vi "test-linear-filter-assert-results.vi"(5 "derivative":i32, 6 "Max":dbl, 7 "Samples":i32, 8 "Min":dbl, 9 "H":dbl, 10 "DerivFunc":refnum<vi>, 11 "F":refnum<vi>) -> (0 "Filt":dbl[](array[numeric]), 1 "Deriv":dbl[](array[numeric]), 2 "Raw":dbl[](array[numeric]), 3 "Passed":bool, 4 "Tolerance":dbl)   [LabVIEW 2019]
uses:
  <vilib>/Rock Robotics/WPI/ThirdParty/JAS_Junk/TrajLib/Matrix_Create.vi
  <vilib>/Rock Robotics/WPI/ThirdParty/JAS_Junk/TrajLib/LinearFilter_Factorial.vi
  <vilib>/Rock Robotics/WPI/ThirdParty/JAS_Junk/TrajLib/LinearFilter_New.vi
  <vilib>/Rock Robotics/WPI/ThirdParty/JAS_Junk/TrajLib/MatBuilder_Create.vi
  <vilib>/gmath/SpecialFunctions.llb/Factorial.vi
  <vilib>/Rock Robotics/SystemInterfaces/NetworkCommunication/NetComm_UsageReport_report.vi
  <vilib>/Analysis/7linalg.llb/Solve Linear Equations.vi
  <vilib>/Analysis/7linalg.llb/Solve Linear Equations (multiple right hand).vi
  <vilib>/Rock Robotics/WPI/ThirdParty/JAS_Junk/TrajLib/Util_LibraryGlobals.vi
  <vilib>/Rock Robotics/WPI/ThirdParty/JAS_Junk/TrajLib/Trajectory_Library.lvlib
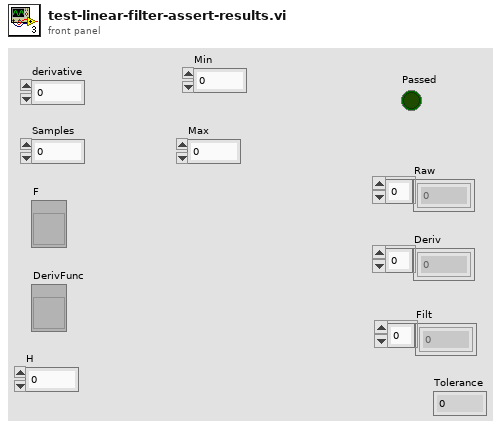
[diagram p1: front panel]
types:
  T1 = typedef "Trajectory_Library.lvlib/LINEAR_FILTER.ctl" = cluster{"InputGains":dbl[], "OutputGains":dbl[], "Inputs":dbl[], "Outputs":dbl[], "InGainCount":i32, "OutGainCount":i32}
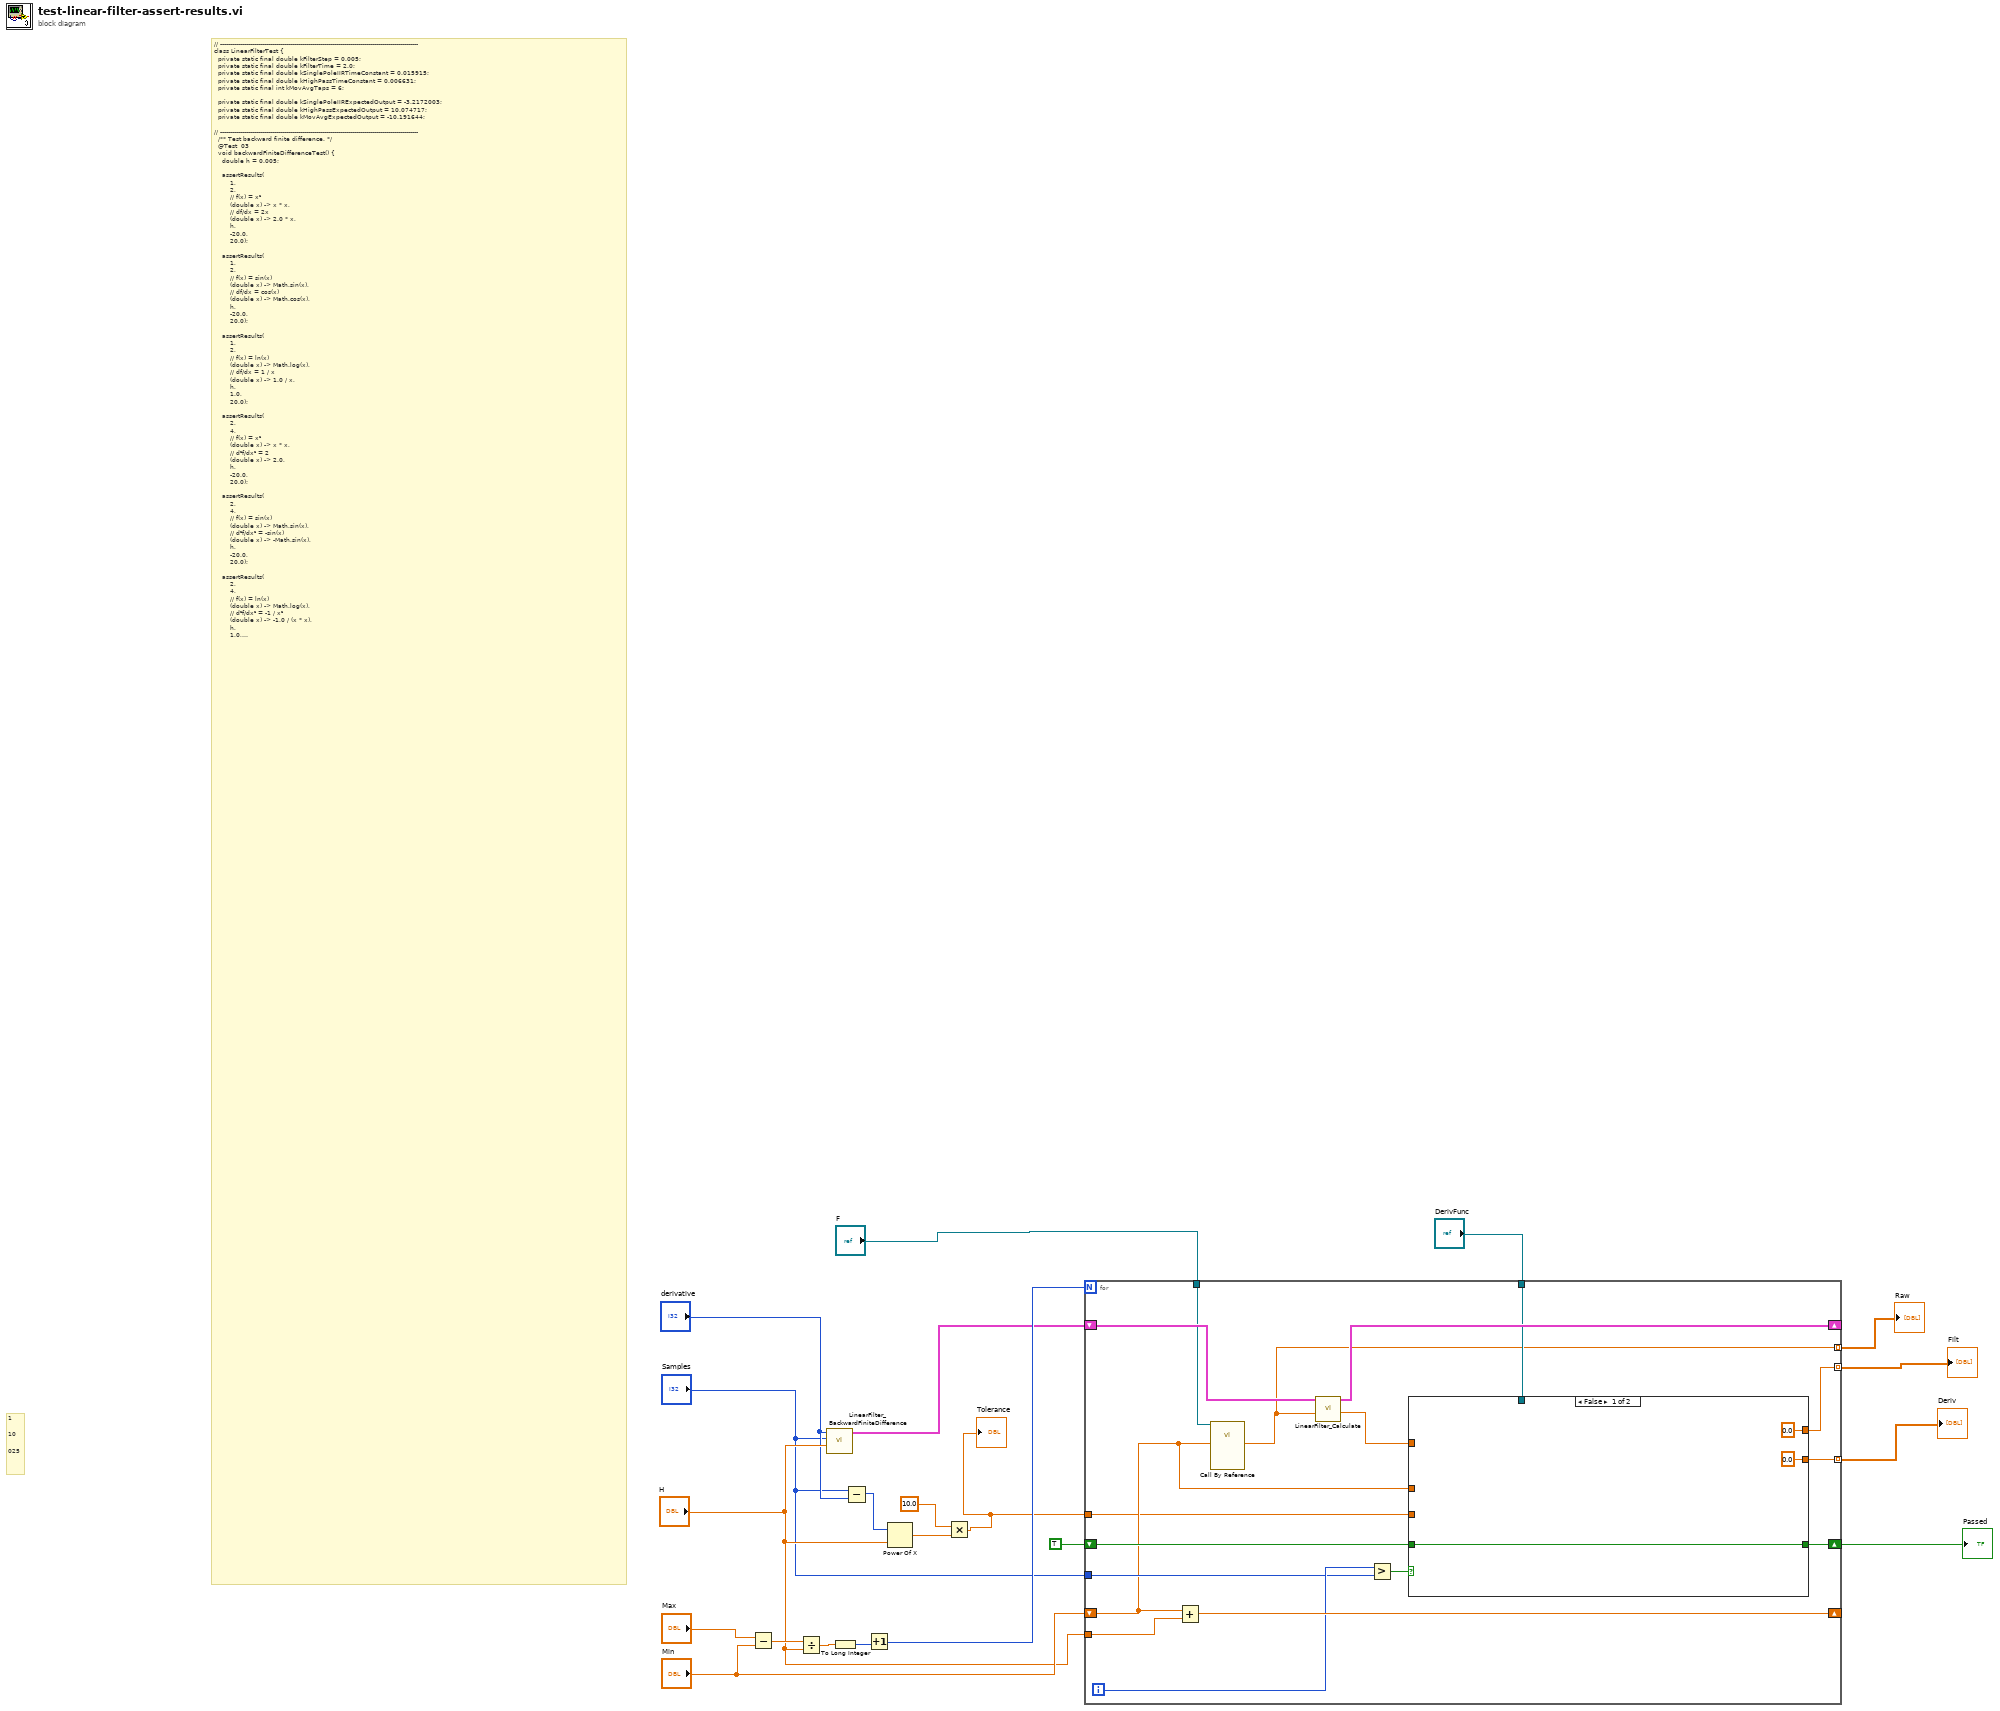
[diagram p0: block diagram]
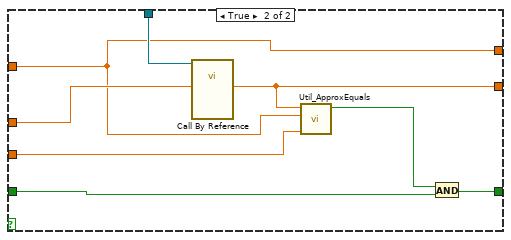
[diagram p2: hidden frame]
diagram:
  # "1\n\n10\n\n025"
  # "// ---------------------------------------------------------------------------------------------------\nclass LinearFilterTest {\n  private static final double kFilterStep = 0.005;\n  private static final double kFilterTime = 2.0;\n  private static final double kSinglePoleIIRTimeConstant = 0.015915;\n  private static final double kHighPassTimeConstant = 0.006631;\n  private static final int kMovAvgTaps = 6;\n\n  private static final double kSinglePoleIIRExpectedOutput = -3.2172003;\n  private static final double kHighPassExpectedOutput = 10.074717;\n  private static final double kMovAvgExpectedOutput = -10.191644;\n\n// ---------------------------------------------------------------------------------------------------\n  /** Test backward finite difference. */\n  @Test  03\n  void backwardFiniteDifferenceTest() {\n    double h = 0.005;\n\n    assertResults(\n        1,\n        2,\n        // f(x) = x²\n        (double x) -> x * x,\n        // df/dx = 2x\n        (double x) -> 2.0 * x,\n        h,\n        -20.0,\n        20.0);\n\n    assertResults(\n        1,\n        2,\n        // f(x) = sin(x)\n        (double x) -> Math.sin(x),\n        // df/dx = cos(x)\n        (double x) -> Math.cos(x),\n        h,\n        -20.0,\n        20.0);\n\n    assertResults(\n        1,\n        2,\n        // f(x) = ln(x)\n        (double x) -> Math.log(x),\n        // df/dx = 1 / x\n        (double x) -> 1.0 / x,\n        h,\n        1.0,\n        20.0);\n\n    assertResults(\n        2,\n        4,\n        // f(x) = x²\n        (double x) -> x * x,\n        // d²f/dx² = 2\n        (double x) -> 2.0,\n        h,\n        -20.0,\n        20.0);\n\n    assertResults(\n        2,\n        4,\n        // f(x) = sin(x)\n        (double x) -> Math.sin(x),\n        // d²f/dx² = -sin(x)\n        (double x) -> -Math.sin(x),\n        h,\n        -20.0,\n        20.0);\n\n    assertResults(\n        2,\n        4,\n        // f(x) = ln(x)\n        (double x) -> Math.log(x),\n        // d²f/dx² = -1 / x²\n        (double x) -> -1.0 / (x * x),\n        h,\n        1.0,\n        20.0);\n  }\n\n// ---------------------------------------------------------------------------------------------------\n  /**\n   * Helper for checking results of backward finite difference.\n   *\n   * @param derivative The order of the derivative.\n   * @param samples The number of sample points.\n   * @param f Function of which to take derivative.\n   * @param dfdx Derivative of f.\n   * @param h Sample period in seconds.\n   * @param min Minimum of f's domain to test.\n   * @param max Maximum of f's domain to test.\n   */\n  void assertResults(\n      int derivative,\n      int samples,\n      DoubleFunction<Double> f,\n      DoubleFunction<Double> dfdx,\n      double h,\n      double min,\n      double max) {\n\n\n    var filter = LinearFilter.backwardFiniteDifference(derivative, samples, h);\n\n    for (int i = (int) (min / h); i < (int) (max / h); ++i) {\n      // Let filter initialize\n      if (i < (int) (min / h) + samples) {\n        filter.calculate(f.apply(i * h));\n        continue;\n      }\n\n      // The order of accuracy is O(h^(N - d)) where N is number of stencil\n      // points and d is order of derivative\n      assertEquals(\n          dfdx.apply(i * h),\n          filter.calculate(f.apply(i * h)),\n          10.0 * Math.pow(h, samples - derivative));\n    }\n  }\n}"
  n1 = Subtract(x="Max", y="Min") -> (x-y=w20:dbl)
  n2 = Divide(x=w20, y="H") -> (x/y=w19:dbl)
  n3 = call <vilib>:"LinearFilter_BackwardFiniteDifference.vi"("Period"="H", "Samples"="Samples", "Derivative"="derivative") -> ("LINEAR_FILTER"=w15:T1)  [unwired: 7 in, 1 out]
  n4 = To Long Integer(number=w19) -> (32bit integer=w18:i32)
  n5 = Subtract(x="Samples", y="derivative") -> (x-y=w9:i32)
  n6 = Increment(x=w18) -> (x+1=w17:i32)
  n7 = Power Of X(1:"H", 2:w9) -> (0:w8:dbl)
  n8 = Multiply(x=10.0, y=w8) -> (x*y=w5:dbl)
  "Tolerance" <- w5
  n9 = for {
    N: w17 -> [_]
    shift-right: [w35] -> _
    shift-left: "Min" -> [w27]
    shift-right: [w37] -> _
    shift-left: w15 -> [w38]
    tunnel: "H" -> [w36]
    tunnel: [w22] -> w3 mode=indexing
    tunnel: "F" -> [w34]
    tunnel: [w26] -> w4 mode=indexing
    tunnel: "Samples" -> [w31]
    shift-right: [w29] -> w12
    shift-left: TRUE -> [w30]
    tunnel: "DerivFunc" -> [w28]
    tunnel: w5 -> [w25]
    tunnel: [w24] -> w2 mode=indexing
    i -> [w32]
    n10 = Add(x=w27, y=w36) -> (x+y=w35:dbl)
    n11 = call-by-ref "?"(reference=w34, "Input"=w27) -> ("Output"=w26:dbl)  [unwired: 11 in, 2 out]
    n12 = call <vilib>:"LinearFilter_Calculate.vi"("Input"=w26, "In LINEAR_FILTER"=w38) -> ("Output"=w23:dbl, "Out LINEAR_FILTER"=w37:T1)  [unwired: 8 in]
    n13 = Greater?(x=w32, y=w31) -> (0:w33:bool)
    n14 = case shown="False" w33 {
      tunnel: w30 -> [w41 w44]
      tunnel: [w41 w46] -> w29
      tunnel: w28 -> [_ w49]
      tunnel: w27 -> [_ w48]
      tunnel: w23 -> [_ w42]
      tunnel: w25 -> [_ w47]
      tunnel: [0.0 ("Output") w43] -> w24
      tunnel: [0.0 ("Output") w42] -> w22
      frame False {
      }
      frame True {
        n15 = call-by-ref "?"(reference=w49, "Input"=w48) -> ("Output"=w43:dbl)  [unwired: 11 in, 2 out]
        n16 = call <vilib>:"Util_ApproxEquals.vi"("Tolerance"=w47, "Value 2"=w42, "Value 1"=w43) -> ("ApproxEquals"=w45:bool)  [unwired: 8 in]
        n17 = And(x=w45, y=w44) -> (x .and. y?=w46:bool)
      }
    }
  }
  "Passed" <- w12
  "Raw" <- w4
  "Filt" <- w3
  "Deriv" <- w2
